vi "CRYGet Operator Window State.vi"(11 "Index":i32) -> (3 "State":bool)   [LabVIEW 2013]
uses:
  CRYWindow/SubVI/CRYMain Sub Window Global.vi
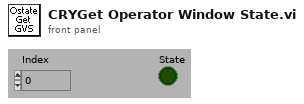
[diagram p1: front panel]
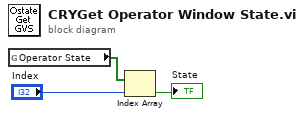
[diagram p0: block diagram]
diagram:
  n1 = global read "CRYMain Sub Window Global.vi" "Operator State"() -> (w2:bool[])
  n2 = Index Array(array=w2, index="Index") -> (element=→"State":bool)
